vi "Get_Tree_Item_Source.vi"(8 "error in (no error)":errorcluster, 11 "IB_TreeSrcItem in":refnum<class "IB_Tree_Item_Source.lvclass">) -> (0 "error out":errorcluster, 3 "IB_TreeSrcItem out":refnum<class "IB_Tree_Item_Source.lvclass">)   [LabVIEW 2020, in "IB_Tree_Item_Source.lvclass"]
uses:
  <vilib>/AppBuilder/IB_Classes/Tree_Item_Source/IB_Tree_Item_Source.lvclass
  <vilib>/AppBuilder/IB_Classes/Tree_Item_Source/IB_Tree_Item_Source.lvclass/IB_Tree_Item_Source.ctl
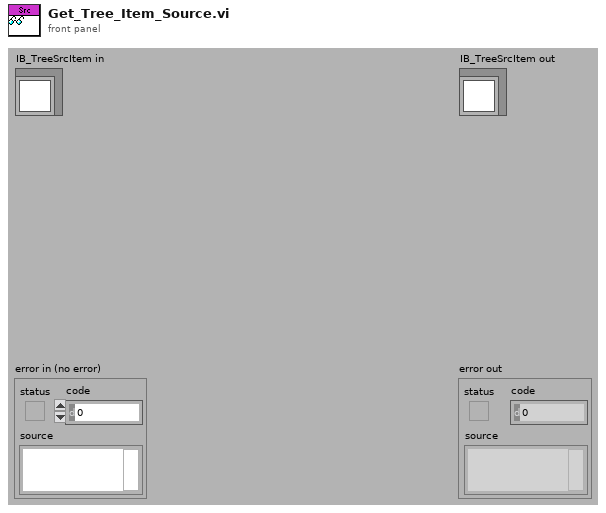
[diagram p1: front panel]
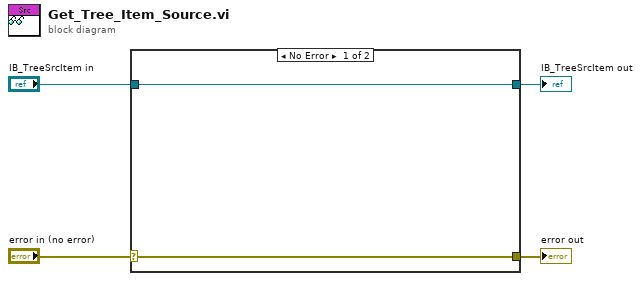
[diagram p0: block diagram]
diagram:
  n1 = case shown="No Error" "error in (no error)" {
    selector: "error in (no error)" -> [w6 w7]
    tunnel: [w6 w7] -> w3
    tunnel: [w5 w8] -> w1
    tunnel: "IB_TreeSrcItem in" -> [w5 w8]
    frame No Error {
    }
    frame Error {
    }
  }
  "error out" <- w3
  "IB_TreeSrcItem out" <- w1
